vi "isDeviceAvailable.vi"(8 "error in (no error)":errorcluster, 10 "device":string, 11 "HWController in":refnum<class "HWController.lvclass">) -> (0 "error out":errorcluster, 2 "available":bool, 3 "HWController out":refnum<class "HWController.lvclass">)   [LabVIEW 2011, in "Hardware.lvlib" / "HWControllers.lvlib" / "HWController.lvclass"]
uses:
  HWController.lvclass
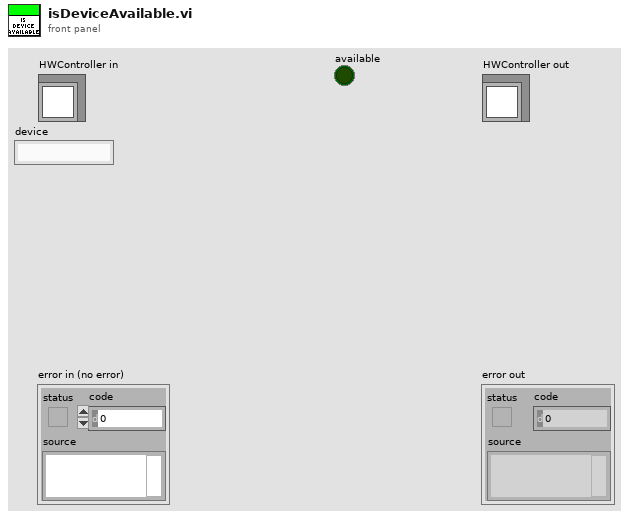
[diagram p1: front panel]
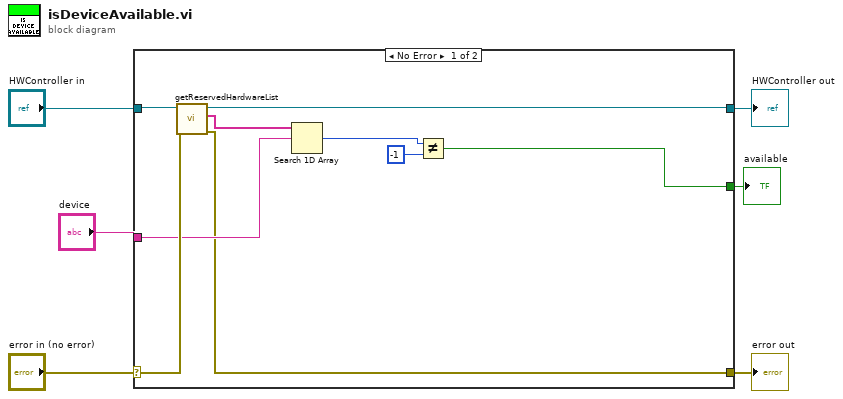
[diagram p0: block diagram]
diagram:
  n1 = case shown="No Error" "error in (no error)" {
    selector: "error in (no error)" -> [w13 w17]
    tunnel: [w7 w17] -> w5
    tunnel: [w14 w16] -> w3
    tunnel: "HWController in" -> [w15 w16]
    tunnel: "device" -> [w11 _]
    tunnel: [w8 _] -> w1
    frame No Error {
      n2 = call "getReservedHardwareList.vi"("error in (no error)"=w13, "HWController.lvclass in"=w15) -> ("error out"=w7:errorcluster, "reservedHardwareList"=w12:string[], "HWController.lvclass out"=w14:refnum<class "HWController.lvclass">)  [unwired: 7 in]
      n3 = Search 1D Array(1D array=w12, element=w11) -> (index of element=w10:i32)  [unwired: 1 in]
      n4 = Not Equal?(x=w10, y=-1) -> (x != y?=w8:bool)
    }
    frame Error {
    }
  }
  "error out" <- w5
  "HWController out" <- w3
  "available" <- w1
